vi "MT EbN0 Calculation(QAM).vi"(0 "Recieved waveform":T3={"t0"=0.0, "dt"=1.0, "Y"=[]} {"Y" format="%.3f"; "dt" format="%^.2e"; "t0" format="%.4f"}, 1 "pulse shaping filter coefficients":dbl[](array[numeric]) format="%.2f", 5 "QAM system parameters":T1={"samples per symbol (16)"=16, "symbol map"=[]} {"symbol map" format="%.3f"}, 7 "synchronization parameters":T2 {"sync sequence" format="%.2f"}, 9 "matched filter coefficients":dbl[](array[numeric]) format="%.2f", 11 "error in (no error)":errorcluster, 12 "reset? (T)":bool=TRUE) -> (4 "Eb/N0":dbl, 6 "Eb/N0(dB)":dbl, 15 "error out":errorcluster)   [LabVIEW 2020, in "niDMT.lvlib"]
uses:
  <vilib>/addons/Modulation/niDMT.lvlib
  <vilib>/addons/Modulation/Analog/controls/Complex Data Waveform.ctl
  <vilib>/Analysis/2dsp.llb/1D Convolution (DBL).vi
  <vilib>/Analysis/NI_AALPro.lvlib
  <vilib>/addons/Modulation/niAMT.lvlib
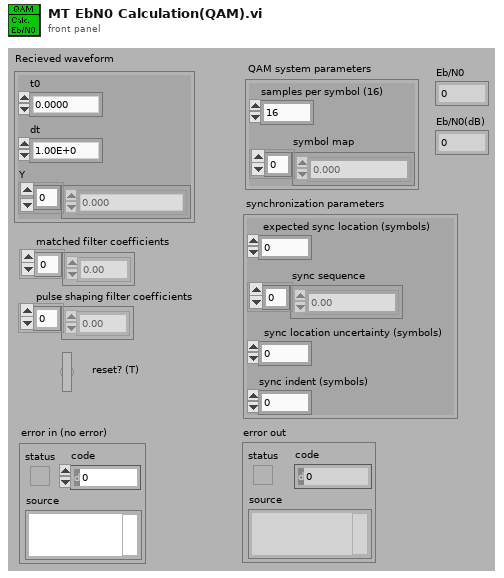
[diagram p1: front panel]
types:
  T1 = cluster{"samples per symbol (16)":i32, "symbol map":cdb[]}
  T2 = cluster{"expected sync location (symbols)":i32, "sync sequence":cdb[], "sync location uncertainty (symbols)":i32, "sync indent (symbols)":i32}
  T3 = typedef "niAMT.lvlib/Complex Data Waveform.ctl" = cluster{"t0":dbl, "dt":dbl, "Y":cdb[]}
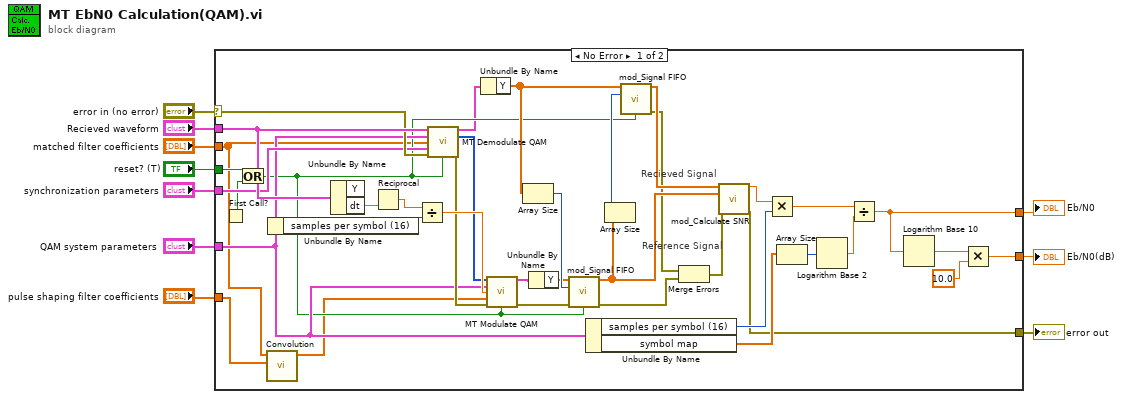
[diagram p0: block diagram]
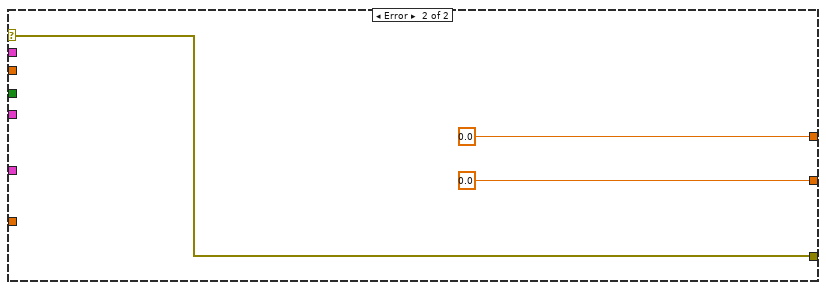
[diagram p2: hidden frame]
diagram:
  n1 = case shown="No Error" "error in (no error)" {
    selector: "error in (no error)" -> [w29 w50]
    tunnel: "pulse shaping filter coefficients" -> [w13 _]
    tunnel: [w38 0.0] -> w9
    tunnel: [w35 0.0] -> w8
    tunnel: "Recieved waveform" -> [w33 _]
    tunnel: "QAM system parameters" -> [w18 _]
    tunnel: "matched filter coefficients" -> [w14 _]
    tunnel: "synchronization parameters" -> [w26 _]
    tunnel: [w19 w50] -> w3
    tunnel: "reset? (T)" -> [w17 _]
    frame No Error {
      # "Recieved Signal"
      # "Reference Signal"
      n2 = First Call?() -> (First Call?: T/F=w16:bool)
      n3 = Or(x=w17, y=w16) -> (x .or. y?=w15:bool)
      n4 = call-poly <vilib>:"Convolution.vi"("Y"=w13, "X"=w14) -> ("X * Y"=w12:dbl[])  [unwired: 1 in, 8 out]
      n5 = Unbundle By Name(w18) -> ("samples per symbol (16)"=w27:i32)
      n6 = Unbundle By Name(w33) -> ("dt"=w49:dbl)  [unwired: 1 out]
      n7 = Reciprocal(x=w49) -> (1/x=w28:dbl)
      n8 = Divide(x=w28, y=w27) -> (x/y=w48:dbl)
      n9 = call <vilib>:"MT Demodulate QAM.vi"("input complex waveform"=w33, "QAM system parameters"=w18, "matched filter coefficients"=w14, "synchronization parameters"=w26, "error in (no error)"=w29, "reset? (T)"=w15) -> ("recovered complex waveform"=w11:T3, "output bit stream"=w44:i8[], "error out"=w32:errorcluster)  [unwired: 1 in, 6 out]
      n10 = Unbundle By Name(w11) -> ("Y"=w30:cdb[])
      n11 = call <vilib>:"MT Modulate QAM.vi"("input bit stream"=w44, "QAM system parameters"=w18, "symbol rate (Hz)"=w48, "pulse shaping filter coefficients"=w12, "error in (no error)"=w32, "reset? (T)"=w15) -> ("output complex waveform"=w34:T3, "error out"=w31:errorcluster)  [unwired: 1 in, 7 out]
      n12 = Array Size(array=w30) -> (size(s)=w42:i32)
      n13 = Unbundle By Name(w34) -> ("Y"=w41:cdb[])
      n14 = call <vilib>:"mod_Signal FIFO.vi"("Signal In"=w41, "Output Length"=w42, "error in (no error)"=w31, "Reset? (T)"=w15) -> ("Signal Out"=w23:cdb[], "error out"=w20:errorcluster)  [unwired: 10 out]
      n15 = Unbundle By Name(w18) -> ("samples per symbol (16)"=w47:i32, "symbol map"=w46:cdb[])
      n16 = Array Size(array=w23) -> (size(s)=w40:i32)
      n17 = call <vilib>:"mod_Signal FIFO.vi"("Signal In"=w30, "Output Length"=w40, "Reset? (T)"=w15) -> ("Signal Out"=w24:cdb[], "error out"=w22:errorcluster)  [unwired: 1 in, 10 out]
      n18 = Merge Errors(w22, w20) -> (w21:errorcluster)
      n19 = call <vilib>:"mod_Calculate SNR.vi"("Recieved Waveform"=w24, "Reference Waveform"=w23, "error in (no error)"=w21) -> ("SNR"=w25:dbl, "error out"=w19:errorcluster)  [unwired: 11 out]
      n20 = Multiply(x=w25, y=w47) -> (x*y=w43:dbl)
      n21 = Array Size(array=w46) -> (size(s)=w45:i32)
      n22 = Logarithm Base 2(1:w45) -> (0:w39:dbl)
      n23 = Divide(x=w43, y=w39) -> (x/y=w38:dbl)
      n24 = Logarithm Base 10(1:w38) -> (0:w37:dbl)
      n25 = Multiply(x=w37, y=10.0) -> (x*y=w35:dbl)
    }
    frame Error {
    }
  }
  "Eb/N0" <- w9
  "Eb/N0(dB)" <- w8
  "error out" <- w3
